vi "initialise.vi"(8 "error in (no error)":errorcluster, 11 "NetworkProEM in":refnum<class "Network_ProEm_WinX32.lvclass">) -> (0 "error out":errorcluster, 3 "NetworkProEM out":refnum<class "Network_ProEm_WinX32.lvclass">)   [LabVIEW 2009, in "Hardware.lvlib" / "HWControllers.lvlib" / "Network_ProEm_WinX32.lvclass"]
uses:
  Network_ProEm_WinX32.lvclass
  Channels/Camera/Camera/Camera.lvclass
  NetworkCamera.lvclass
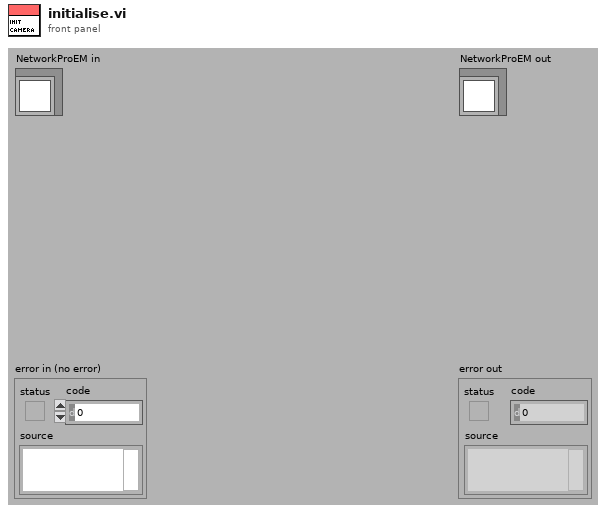
[diagram p1: front panel]
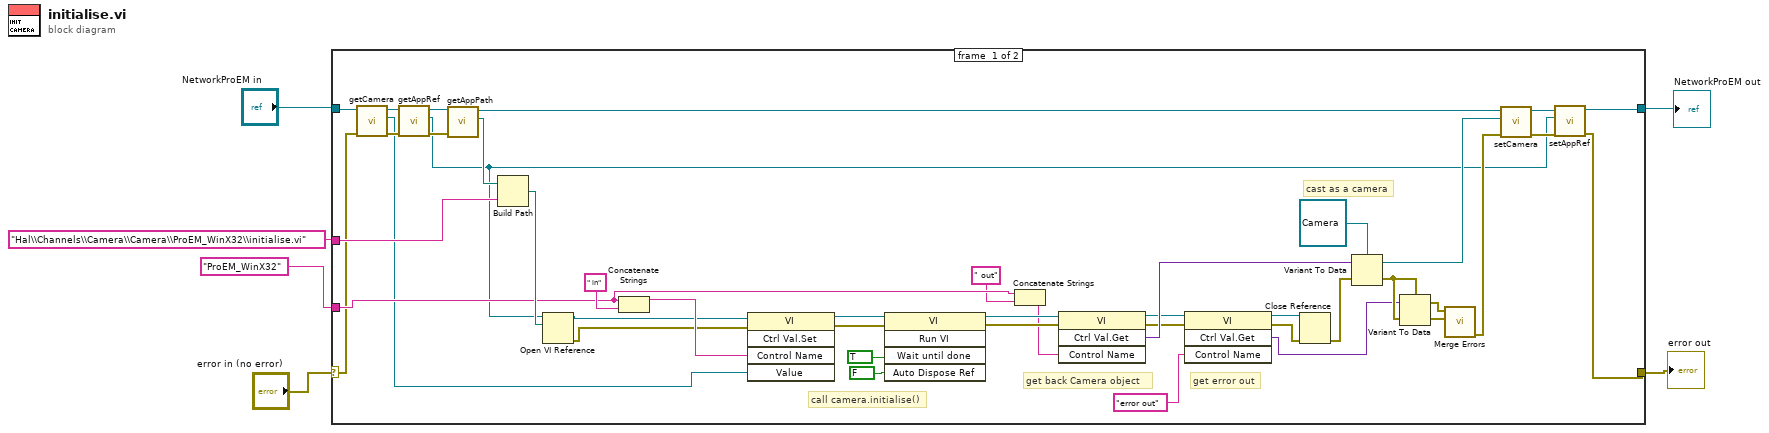
[diagram p0: block diagram]
diagram:
  n1 = case shown="No Error" "error in (no error)" {
    selector: "error in (no error)" -> [w14 w51]
    tunnel: [w26 w51] -> w2
    tunnel: [w30 w50] -> w1
    tunnel: "NetworkProEM in" -> [w33 w50]
    tunnel: "Hal\\Channels\\Camera\\Camera\\ProEM_WinX32\\initialise.vi" ("viPath") -> [w39 _]
    tunnel: "ProEM_WinX32" ("Control name") -> [w36 _]
    frame #0 {
      # "get error out"
      # "get back Camera object"
      # "call camera.initialise()"
      # "cast as a camera"
      n2 = call "getCamera.vi"("error in (no error)"=w14, "NetworkCamera in"=w33) -> ("error out"=w16:errorcluster, "Camera"=w9:refnum<class "Camera.lvclass">, "NetworkCamera out"=w32:refnum<class "Network_ProEm_WinX32.lvclass">)  [unwired: 7 in]
      n3 = call "getAppRef.vi"("error in (no error)"=w16, "NetworkCamera in"=w32) -> ("error out"=w15:errorcluster, "appRef"=w11:refnum<vi>, "NetworkCamera out"=w31:refnum<class "Network_ProEm_WinX32.lvclass">)  [unwired: 7 in]
      n4 = call "getAppPath.vi"("error in (no error)"=w15, "NetworkCamera in"=w31) -> ("appPath"=w12:path, "NetworkCamera out"=w29:refnum<class "Network_ProEm_WinX32.lvclass">)  [unwired: 7 in, 1 out]
      n5 = Build Path(base path=w12, name or relative path=w39) -> (appended path=w49:path)
      n6 = Open VI Reference(application reference (local)=w11, vi path=w49) -> (vi reference=w8:refnum<vi>, error out=w7:errorcluster)  [unwired: 4 in]
      n7 = Concatenate Strings(w36, " in") -> (w37:string)
      n8 = invoke class="VI" method="Ctrl Val.Set"(reference=w8, error in=w7, "Control Name"=w37, "Value"=w9) -> (reference out=w48:refnum<vi>, error out=w47:errorcluster)  [unwired: 1 in, 3 out]
      n9 = invoke class="VI" method="Run VI"(reference=w48, error in=w47, "Wait until done"=TRUE, "Auto Dispose Ref"=FALSE) -> (reference out=w45:refnum<vi>, error out=w44:errorcluster)  [unwired: 1 in, 3 out]
      n10 = Concatenate Strings(w36, " out") -> (w34:string)
      n11 = invoke class="VI" method="Ctrl Val.Get"(reference=w45, error in=w44, "Control Name"=w34) -> (reference out=w41:refnum<vi>, error out=w23:errorcluster, "Get Control Value Variant"=w42:variant)  [unwired: 1 in, 1 out]
      n12 = invoke class="VI" method="Ctrl Val.Get"(reference=w41, error in=w23, "Control Name"="error out") -> (reference out=w24:refnum<vi>, error out=w10:errorcluster, "Get Control Value Variant"=w21:variant)  [unwired: 1 in, 1 out]
      n13 = Close Reference(reference=w24, error in (no error)=w10) -> (error out=w40:errorcluster)
      n14 = Variant To Data(error in=w40, Variant=w42, type=refnum<class "Camera.lvclass"> refnum ("Camera out")) -> (error out=w22:errorcluster, data=w28:refnum<class "Camera.lvclass">)
      n15 = Variant To Data(error in=w22, Variant=w21, type=w22) -> (error out=w20:errorcluster, data=w19:errorcluster)
      n16 = call <vilib>:"Merge Errors.vi"("error in 2 (no error)"=w20, "error in 1 (no error)"=w19) -> ("error out"=w18:errorcluster)  [unwired: 5 in]
      n17 = call "setCamera.vi"("error in (no error)"=w18, "Camera"=w28, "NetworkCamera in"=w29) -> ("error out"=w25:errorcluster, "NetworkCamera out"=w27:refnum<class "Network_ProEm_WinX32.lvclass">)  [unwired: 7 in]
      n18 = call "setAppRef.vi"("error in (no error)"=w25, "appRef"=w11, "NetworkCamera in"=w27) -> ("error out"=w26:errorcluster, "NetworkCamera out"=w30:refnum<class "Network_ProEm_WinX32.lvclass">)  [unwired: 7 in]
    }
    frame #1 {
    }
  }
  "error out" <- w2
  "NetworkProEM out" <- w1
